vi "ag33xxx - Catalog.vi"(8 "error in (no error)":errorcluster, 10 "Location (F: User-Defined)":bool, 11 "VISA session":refnum<visa-resource-name>) -> (0 "error out":errorcluster, 2 "Catalog":string, 3 "dup VISA session":refnum<visa-resource-name>)   [LabVIEW 2014, in "AG33XXX.lvlib"]
doc: "Outputs the list of the names of arbitrary waveforms currently uploaded to the instrument's memory.\n\nThis is an adapted VI that should, in principe, be part of the instrument driver. However, I do not like to patch the original driver. This this VI has been added to the library of the CS class."
uses:
  AG33XXX.lvlib
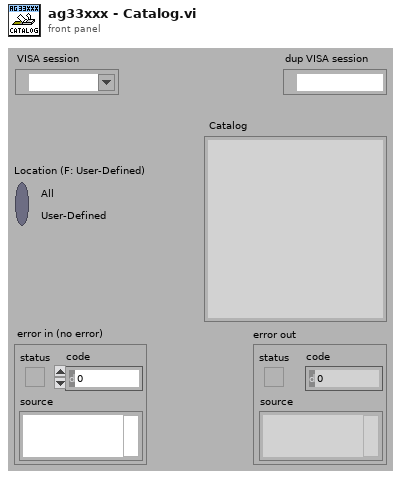
[diagram p1: front panel]
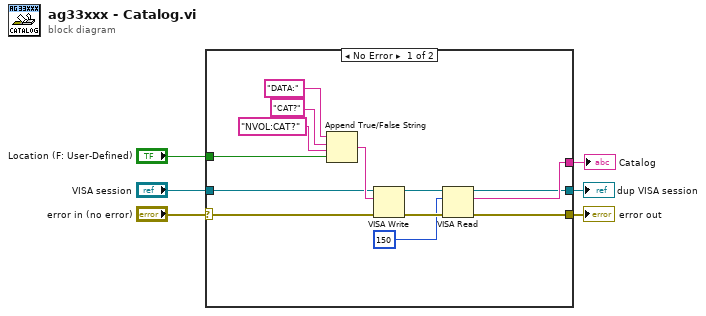
[diagram p0: block diagram]
diagram:
  n1 = case shown="No Error" "error in (no error)" {
    selector: "error in (no error)" -> [w7 w20]
    tunnel: "Location (F: User-Defined)" -> [w15 _]
    tunnel: [w14 _] -> w5
    tunnel: [w13 w20] -> w4
    tunnel: [w9 w21] -> w3
    tunnel: "VISA session" -> [w8 w21]
    frame No Error {
      n2 = Append True/False String(1:w15, 2:"NVOL:CAT?", 3:"CAT?", 4:"DATA:") -> (0:w19:string)
      n3 = VISA Write(VISA resource name=w8, write buffer=w19, error in (no error)=w7) -> (VISA resource name out=w10:refnum<visa-resource-name>, error out=w12:errorcluster)  [unwired: 1 out]
      n4 = VISA Read(VISA resource name=w10, byte count=u32 150, error in (no error)=w12) -> (VISA resource name out=w9:refnum<visa-resource-name>, read buffer=w14:string, error out=w13:errorcluster)  [unwired: 1 out]
    }
    frame Error {
    }
  }
  "error out" <- w4
  "Catalog" <- w5
  "dup VISA session" <- w3
